vi "Set File Properties.vi"(8 "error in (no error)":errorcluster, 10 "File":T1, 11 "CubeLogger in":refnum<class "CubeLogger.lvclass">) -> (0 "error out":errorcluster, 2 "Canceled?":bool, 3 "CubeLogger out":refnum<class "CubeLogger.lvclass">)   [LabVIEW 2018, in "CubeLogger.lvclass"]
uses:
  CubeLogger.lvclass
  File.ctl
  CubeLogger.lvclass/CubeLogger.ctl
panel:
  out "Canceled?":bool
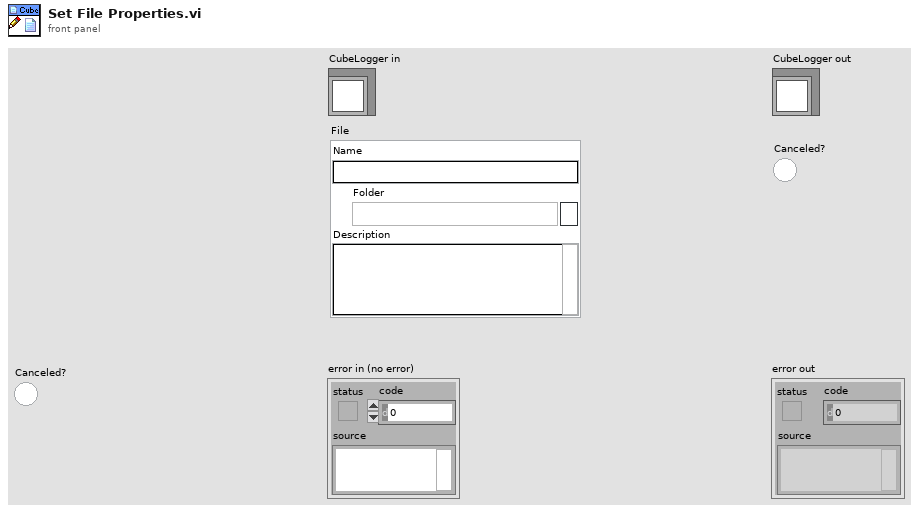
[diagram p1: front panel]
types:
  T1 = typedef "CubeLogger.lvclass/File.ctl" = cluster{"Name":string, "Folder":path, "Description":string}
  T2 = enum16{"open", "replace", "create", "open or create", "replace or create", "replace or create with confirmation"}
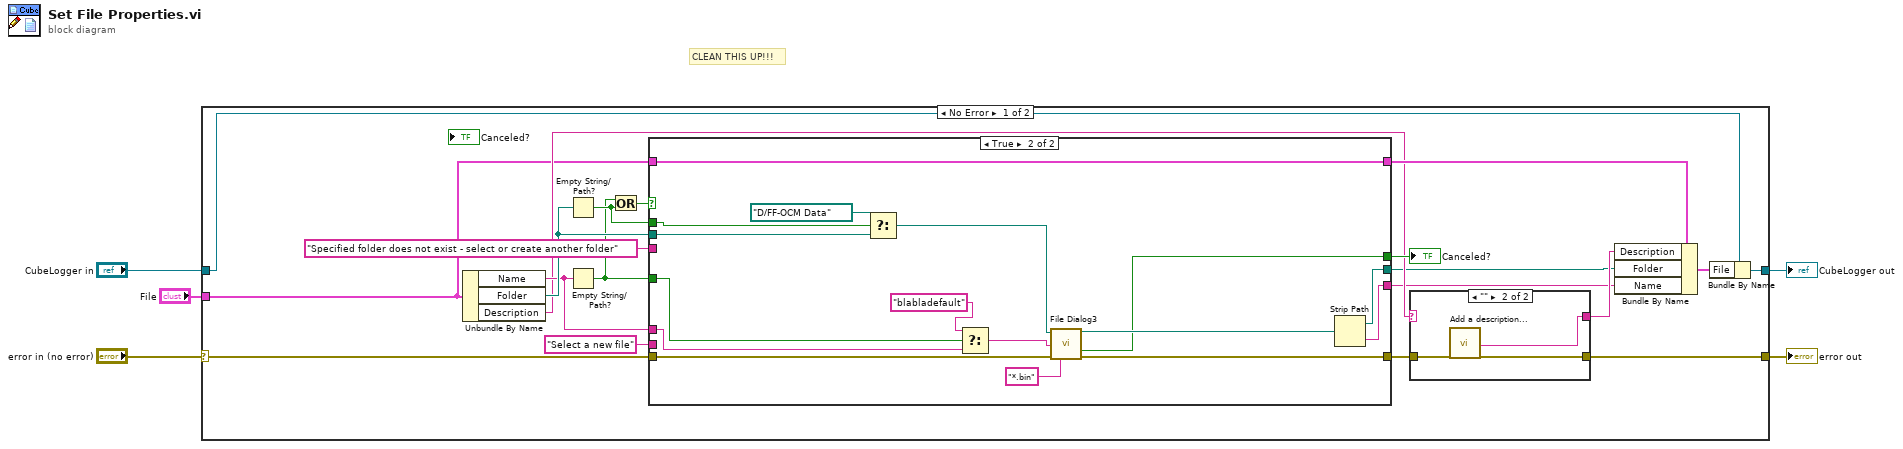
[diagram p0: block diagram]
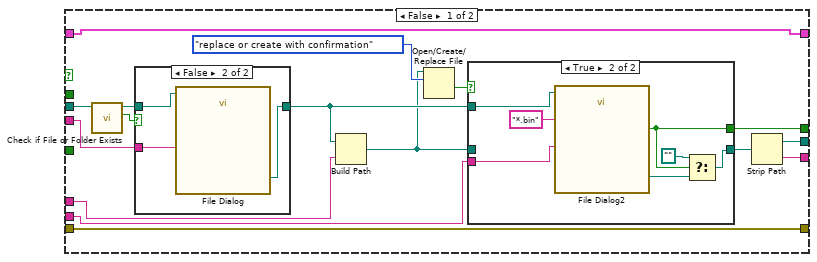
[diagram p3: hidden frame]
diagram:
  # "CLEAN THIS UP!!!"
  n1 = case shown="No Error" "error in (no error)" {
    selector: "error in (no error)" -> [w10 w76]
    tunnel: [w9 w76] -> w4
    tunnel: [w7 w75] -> w2
    tunnel: "CubeLogger in" -> [w8 w75]
    tunnel: "File" -> [w11 _]
    frame No Error {
      n2 = Unbundle By Name(w11) -> ("Name"=w19:string, "Folder"=w21:path, "Description"=w17:string)
      n3 = Empty String/Path?(string/path=w21) -> (empty?=w22:bool)
      n4 = Empty String/Path?(string/path=w19) -> (empty?=w20:bool)
      n5 = Or(x=w20, y=w22) -> (x .or. y?=w25:bool)
      n6 = case shown="True" w25 {
        tunnel: [w46 w74] -> w24
        tunnel: w11 -> [w46 w74]
        tunnel: [w32 w68] -> w23
        tunnel: w22 -> [_ w73]
        tunnel: w21 -> [w41 w72]
        tunnel: w20 -> [_ w66]
        tunnel: w19 -> [w40 w65]
        tunnel: w10 -> [w45 w63]
        tunnel: [w45 w62] -> w18
        tunnel: "Specified folder does not exist - select or create another folder" -> [w42 _]
        tunnel: "Select a new file" -> [w36 _]
        tunnel: [w34 w61] -> w13
        tunnel: [w33 w60] -> w12
        frame False {
          n7 = call <vilib>:"Check if File or Folder Exists.vi"("path"=w41) -> ("file or folder exists?"=w43:bool, "dup path"=w44:path)  [unwired: 8 in, 1 out]
          n8 = case shown="False" w43 {
            tunnel: w44 -> [w55 w58]
            tunnel: [w55 w57] -> w38
            tunnel: w42 -> [_ w56]
            frame True {
            }
            frame False {
              n9 = call "File Dialog"("start path"=w58, "prompt"=w56) -> ("selected path"=w57:path)  [unwired: 10 in, 3 out]
            }
          }
          n10 = Build Path(base path=w38, name or relative path=w40) -> (appended path=w31:path)
          n11 = Open/Create/Replace File(file path (use dialog)=w31, operation (0:open)=T2."replace or create with confirmation") -> (cancelled=w37:bool)  [unwired: 4 in, 2 out]
          n12 = case shown="True" w37 {
            tunnel: w38 -> [_ w54]
            tunnel: [w47 w49] -> w35
            tunnel: w36 -> [_ w53]
            tunnel: [_ w51] -> w32
            tunnel: w31 -> [w47 _]
            frame False {
            }
            frame True {
              n13 = call "File Dialog2"("start path"=w54, "prompt"=w53, "pattern (all files)"="*.bin") -> ("selected path"=w50:path, "cancelled"=w51:bool)  [unwired: 9 in, 2 out]
              n14 = Select(t=path "", s=w51, f=w50) -> (s? t:f=w49:path)
            }
          }
          n15 = Strip Path(path=w35) -> (stripped path=w34:path, name=w33:string)
        }
        frame True {
          n16 = Select(t=path "D:/FF-OCM Data", s=w73, f=w72) -> (s? t:f=w70:path)
          n17 = Select(t="blabladefault", s=w66, f=w65) -> (s? t:f=w64:string)
          n18 = call "File Dialog3"("start path"=w70, "default name"=w64, "error in"=w63, "pattern (all files)"="*.bin") -> ("selected path"=w69:path, "cancelled"=w68:bool, "error out"=w62:errorcluster)  [unwired: 8 in, 1 out]
          n19 = Strip Path(path=w69) -> (stripped path=w61:path, name=w60:string)
        }
      }
      "Canceled?" <- w23
      n20 = case shown="\"\"" w17 {
        selector: w17 -> [w26 _]
        tunnel: [w27 w30] -> w9
        tunnel: w18 -> [w27 w29]
        tunnel: [w26 w28] -> w16
        frame Default {
        }
        frame "" {
          n21 = call "Add a description..."("error in (no error)"=w29) -> ("Description"=w28:string, "error out"=w30:errorcluster)  [unwired: 16 in, 1 out]
        }
      }
      n22 = Bundle By Name(cluster=w24, "Description"=w16, "Folder"=w13, "Name"=w12) -> (w6:T1)
      n23 = Bundle By Name(cluster=w8, "File"=w6) -> (w7:refnum<class "CubeLogger.lvclass">)
    }
    frame Error {
    }
  }
  "error out" <- w4
  "CubeLogger out" <- w2
